vi "CreateNewFile.vi"(7 "TriggerTimeStamp":timestamp=timestamp(3569548862.6211414 s since 1904-01-01), 8 "error in (no error)":errorcluster, 10 "Data":waveform(dbl)[](array[waveform]), 11 "Logging Configuration":T1={"Log File Base Path"=path "", "Samples to Save"=0, "Trigger - Threshold"=0.0, "Trigger - Channel"=0, "Always Log"=FALSE, "External Trigger"=FALSE, "External Trigger Armed"=FALSE, "TDMS File Reference"=refnum, "DAQVersion"="", "SWVersion"="", "CircSamples"=0, "BeepWhenComplete"=FALSE, "ChannelConfig"=[], "ActiveChannels"=[], "Title"="", "Description"="", "ChannelNames"=[], "ResponseExtension"=TRUE}) -> (0 "error out":errorcluster, 3 "Logging Config Out":T1={"Log File Base Path"=path "", "Samples to Save"=0, "Trigger - Threshold"=0.0, "Trigger - Channel"=0, "Always Log"=FALSE, "External Trigger"=FALSE, "External Trigger Armed"=FALSE, "TDMS File Reference"=refnum, "DAQVersion"="", "SWVersion"="", "CircSamples"=0, "BeepWhenComplete"=FALSE, "ChannelConfig"=[], "ActiveChannels"=[], "Title"="", "Description"="", "ChannelNames"=[], "ResponseExtension"=TRUE})   [LabVIEW 2017, in "Logging.lvlib"]
uses:
  Logging.lvlib
  Logging Configuration.ctl
  <vilib>/Analysis/baseanly.llb/Mean (DBL).vi
  <vilib>/Analysis/NI_AALBase.lvlib
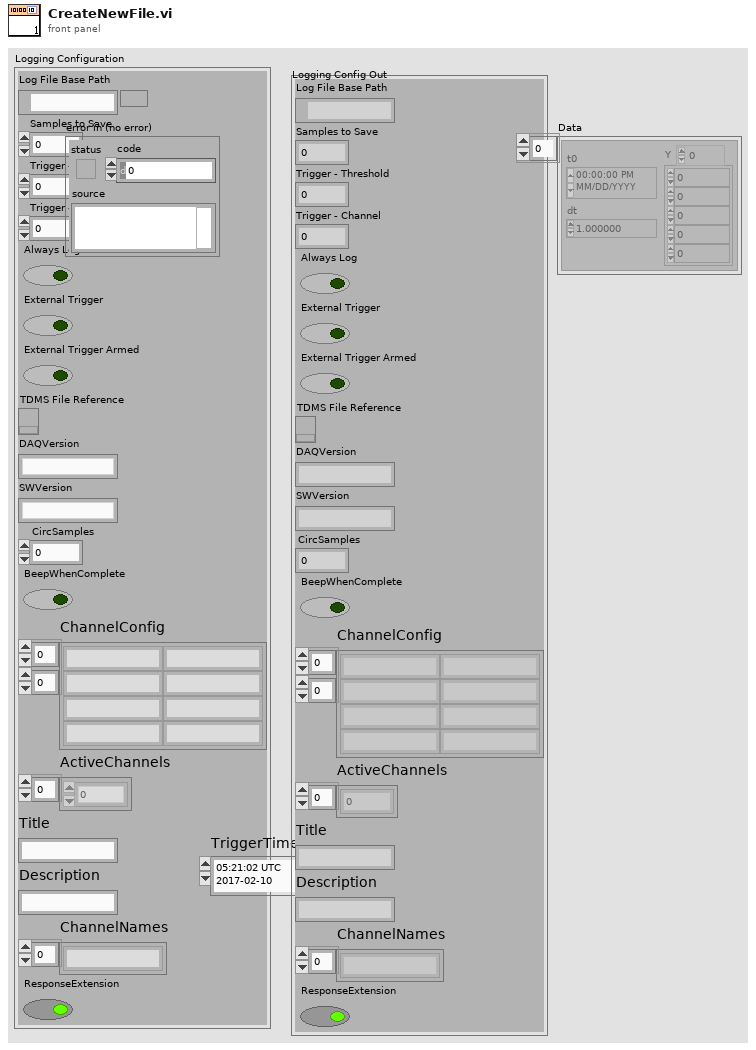
[diagram p1: front panel]
types:
  T1 = typedef "Logging.lvlib/Logging Configuration.ctl" = cluster{"Log File Base Path":path, "Samples to Save":u32, "Trigger - Threshold":dbl, "Trigger - Channel":u32, "Always Log":bool, "External Trigger":bool, "External Trigger Armed":bool, "TDMS File Reference":refnum<k34>, "DAQVersion":string, "SWVersion":string, "CircSamples":u32, "BeepWhenComplete":bool, "ChannelConfig":string[][], "ActiveChannels":i32[], "Title":string, "Description":string, "ChannelNames":string[], "ResponseExtension":bool}
  T2 = enum16{"open", "open or create", "create or replace", "create", "open (read-only)"}
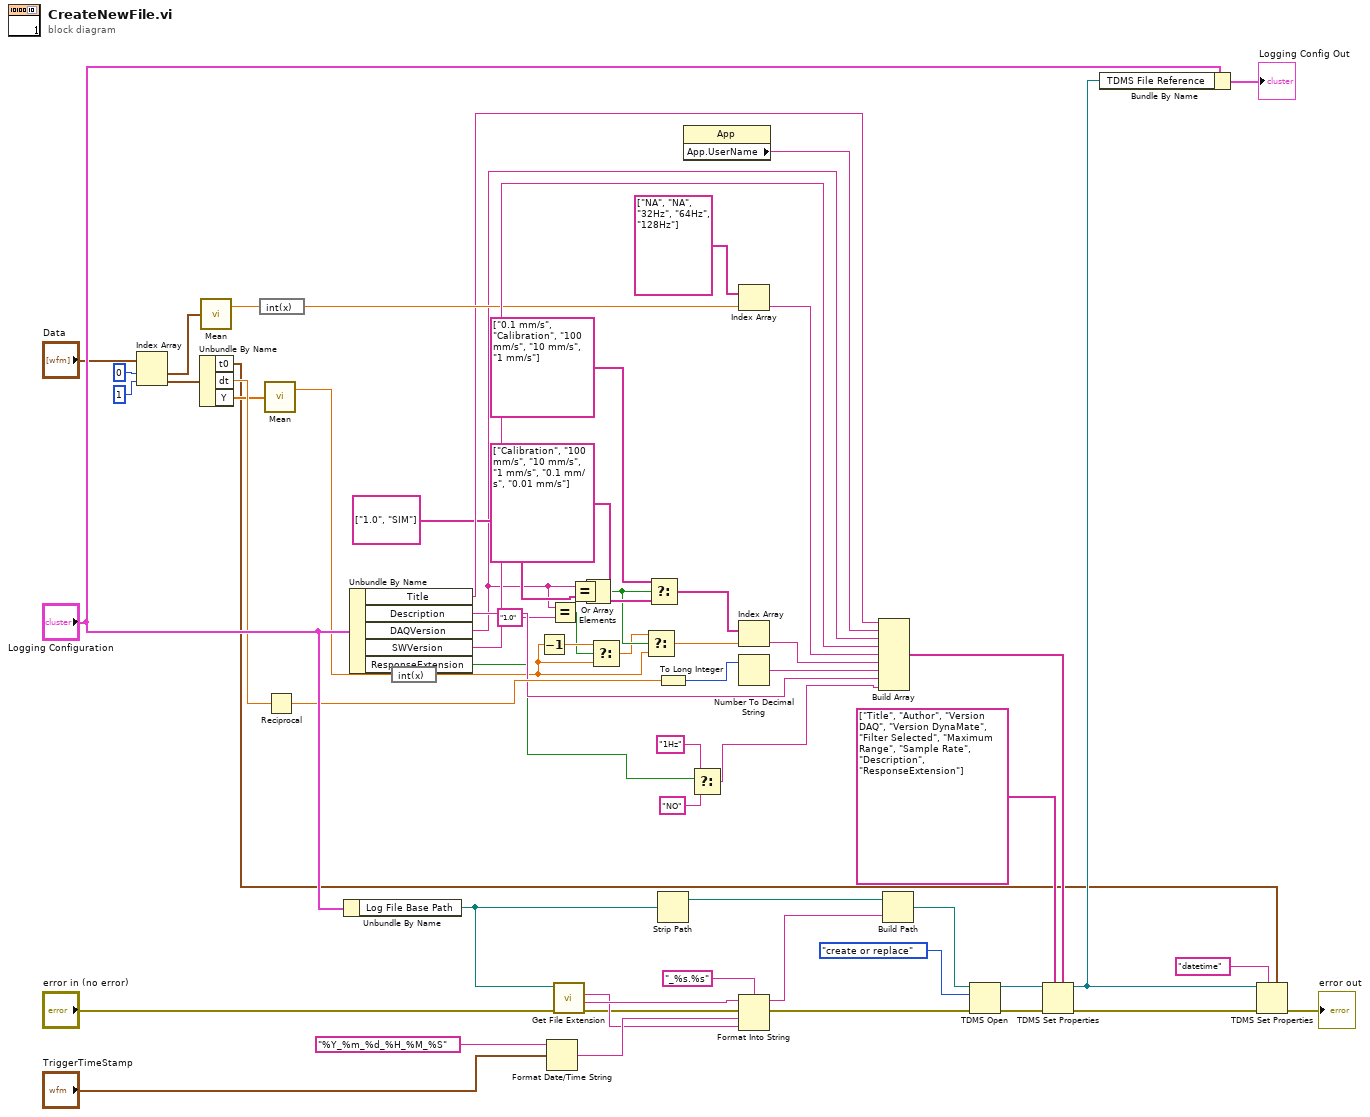
[diagram p0: block diagram]
diagram:
  n1 = Index Array(array="Data", index #1=0 ("index"), index #2=1 ("index")) -> (element #1=w34:waveform(dbl), element #2=w26:waveform(dbl))
  n2 = Unbundle By Name(w26) -> ("t0"=w16:timestamp, "dt"=w25:dbl, "Y"=w21:dbl[])
  n3 = call-poly <vilib>:"Mean.vi"("X"=w34) -> ("mean"=w35:dbl)  [unwired: 1 out]
  n4 = expression code="int(x)"(w35) -> (w32:dbl)
  n5 = call-poly <vilib>:"Mean.vi"("X"=w21) -> ("mean"=w39:dbl)  [unwired: 1 out]
  n6 = Reciprocal(x=w25) -> (1/x=w24:dbl)
  n7 = Unbundle By Name("Logging Configuration") -> ("Log File Base Path"=w59:path)
  n8 = Unbundle By Name("Logging Configuration") -> ("Title"=w20:string, "Description"=w17:string, "DAQVersion"=w10:string, "SWVersion"=w49:string, "ResponseExtension"=w4:bool)
  n9 = expression code="int(x)"(w39) -> (w6:dbl)
  n10 = Decrement(x=w6) -> (x-1=w8:dbl)
  n11 = Format Date/Time String(time format string (%c)="%Y_%m_%d_%H_%M_%S", seconds (now)="TriggerTimeStamp") -> (date/time string=w56:string)  [unwired: 1 in]
  n12 = Equal?(x=w10, y="1.0") -> (x = y?=w5:bool)
  n13 = call <vilib>:"Get File Extension.vi"("error in (no error)"="error in (no error)", "file"=w59) -> ("error out"=w47:errorcluster, "filename without extension"=w57:string, "lowercase file extension"=w55:string)  [unwired: 5 in, 2 out]
  n14 = Equal?(x=w10, y=string[] ["1.0", "SIM"]) -> (x = y?=w30:bool[])
  n15 = Or Array Elements(Boolean array=w30) -> (logical OR=w11:bool)
  n16 = Select(t=w8, s=w5, f=w6) -> (s? t:f=w7:dbl)
  n17 = Select(t=w7, s=w11, f=w6) -> (s? t:f=w28:dbl)
  n18 = Select(t=string[] ["0.1 mm/s", "Calibration", "100 mm/s", "10 mm/s", "1 mm/s"], s=w11, f=string[] ["Calibration", "100 mm/s", "10 mm/s", "1 mm/s", "0.1 mm/s", "0.01 mm/s"]) -> (s? t:f=w29:string[])
  n19 = To Long Integer(number=w24) -> (32bit integer=w22:i32)
  n20 = Strip Path(path=w59) -> (stripped path=w58:path)  [unwired: 1 out]
  n21 = property class="App"() -> ("App.UserName"=w51:string)  [unwired: 2 in, 2 out]
  n22 = Select(t="1Hz", s=w4, f="NO") -> (s? t:f=w3:string)
  n23 = Index Array(array=string[] ["NA", "NA", "32Hz", "64Hz", "128Hz"], index=w32) -> (element=w31:string)
  n24 = Index Array(array=w29, index=w28) -> (element=w27:string)
  n25 = Number To Decimal String(number=w22) -> (decimal integer string=w23:string)  [unwired: 1 in]
  n26 = Format Into String(format string="_%s.%s", initial string=w57, error in=w47, w56, w55) -> (resulting string=w54:string, error out=w46:errorcluster)
  n27 = Build Array(w20, w51, w10, w49, w31, w27, w23, w17, w3) -> (w50:string[])
  n28 = Build Path(base path=w58, name or relative path=w54) -> (appended path=w53:path)
  n29 = TDMS Open(8:w46, 10:T2."create or replace" ("operation (0:open)"), 11:w53) -> (0:w45:errorcluster, 3:w18:refnum<k34>)  [unwired: 4 in]
  n30 = TDMS Set Properties(5:w50, 7:string[] ["Title", "Author", "Version DAQ", "Version DynaMate", "Filter Selected", "Maximum Range", "Sample Rate", "Description", "ResponseExtension"] ("property names"), 8:w45, 11:w18) -> (0:w14:errorcluster, 3:w19:refnum<k34>)  [unwired: 4 out]
  n31 = Bundle By Name(cluster="Logging Configuration", "TDMS File Reference"=w19) -> (→"Logging Config Out":T1)
  n32 = TDMS Set Properties(5:w16, 7:"datetime", 8:w14, 11:w19) -> (0:→"error out":errorcluster)  [unwired: 5 out]
